vi "ABOUT.vi"() -> ()   [LabVIEW 2015]
uses:
  Controls/FGV_Options.ctl
  Controls/HID State.ctl
panel:
  out "Demo SubTitle":string
  out "Demo Title":string
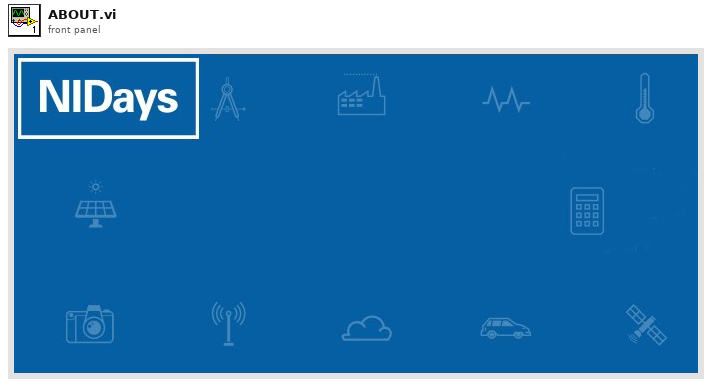
[diagram p1: front panel]
types:
  T1 = typedef "FGV_Options.ctl" = enum16{"Read from File", "Write to File", "Get", "Set"}
  T2 = typedef "HID Data.ctl" = cluster{"IMAQdx Session":T3, "Resampled Image":T4, "Low Level Grab":T4, "X Resolution":i32, "Y Resolution":i32, "Image Threshold":u8, "Reset Value":i32, "FIFO Timer":u16, "Row Timer":u32, "Memory Writer Timer":u8, "Color":enum16{"Green", "Blue", "Red", "White", "Pink", "Yellow", "Turquoise", "Black"}, "Top":bool[][], "Bottom":bool[][], "Timeout (ms)":i32, "Menu Tag":string, "Color Background":enum16{"Green", "Blue", "Red", "White", "Pink", "Yellow", "Turquoise", "Black"}, "FPGA VI Reference":refnum<k20>, "Next Steps":T5[], "Turn off LED Matrix":bool, "FPGA Alias":string, "FPGA Bitfile":path, "Localized Texts":cluster{"Status Text":cluster{"Status Text Table":string[], "Status Text Index":i32}, "Controls":cluster{"Control Text Table":string[], "Control Text Index":i32}, "Titles":cluster{"Titles Text Table":string[], "Titles Text Index":i32}}, "Language":u16}
  T3 = typedef "IMAQdx.ctl" = refnum<k21>
  T4 = typedef "IMAQ Image.ctl" = refnum<image>
  T5 = typedef "HID State.ctl" = enum16{"Initialize", "Set FPGA Parametes", "Set Camera Parameters", "Set LED Matrix Parameters", "Initialize FPGA Interface", "Initialize Camera", "Start FPGA VI", "Start Camera", "Wait for Event", "Update UI", "Acquire", "Process Image", "Get Boolean Arrays", "Send to FPGA", "Menu Pop-Up", "Menu Actions", "Handle Errors", "Close Camera", "Close FPGA", "Stop", "Exit"}
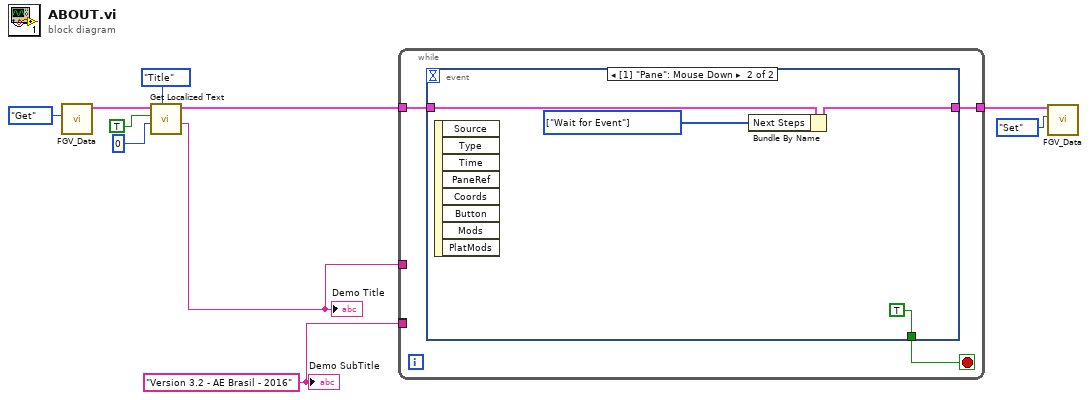
[diagram p0: block diagram]
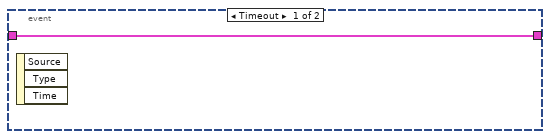
[diagram p2: hidden frame]
diagram:
  w7 = "Version 3.2 - AE Brasil - 2016" ("Demo SubTitle")
  n1 = call "FGV_Data.vi"("Option"=FGV_Options."Get") -> ("Data Out"=w5:T2)  [unwired: 9 in, 1 out]
  n2 = call "Get Localized Text.vi"("Text Type"=enum16{"Status", "Title", "Controls"}."Title", "Text Index"=0, "Force Index"=TRUE, "Data In"=w5) -> ("Localized Text"=w6:string, "Data Out"=w4:T2)  [unwired: 6 in]
  "Demo Title" <- w6
  n3 = while {
    tunnel: w4 -> [w13]
    tunnel: [w12] -> w8
    tunnel: w6 -> [_]
    tunnel: [w11] -> _
    tunnel: w7 -> [w11]
    stop <- w14 stop-if-true
    n4 = event shown="[1] \"Pane\": Mouse Down" {
      selector: _ -> [_ _]
      dyn-events: _ -> [_ _]
      timeout: _ -> [_ _]
      tunnel: [_ TRUE] -> w14
      tunnel: w13 -> [w15 w18]
      tunnel: [w15 w17] -> w12
      event Timeout {
        n5 = event-data() -> ()  [unwired: 1 in, 3 out]
      }
      event Mouse Down {
        w16 = T5[] [enum."Wait for Event"] items=["Initialize", "Set FPGA Parametes", "Set Camera Parameters", "Set LED Matrix Parameters", "Initialize FPGA Interface", "Initialize Camera", "Start FPGA VI", "Start Camera", "Wait for Event", "Update UI", "Acquire", "Process Image", "Get Boolean Arrays", "Send to FPGA", "Menu Pop-Up", "Menu Actions", "Handle Errors", "Close Camera", "Close FPGA", "Stop", "Exit"] ("Array")
        n6 = event-data() -> ()  [unwired: 1 in, 8 out]
        n7 = Bundle By Name(cluster=w18, "Next Steps"=w16) -> (w17:T2)
      }
    }
  }
  n8 = call "FGV_Data.vi"("Option"=FGV_Options."Set", "Data In"=w8) -> ()  [unwired: 8 in, 2 out]
  "Demo SubTitle" <- w7
